vi "控件拖动.vi"() -> ()   [LabVIEW 2016]
uses:
  <vilib>/Utility/miscctls.llb/LVPointTypeDef.ctl
  <vilib>/Utility/miscctls.llb/LVPositionTypeDef.ctl
panel:
  in  "供电模块":T1 {"蓄电池2"."电量" format="%.0f %"; "蓄电池2"."电池电量" scale=0.0..100.0; "蓄电池2"."电流" format="%#.2g"; "蓄电池2"."电压" format="%#.2g"; "蓄电池"."电量" format="%.0f %"; "蓄电池"."电池电量" scale=0.0..100.0; "蓄电池"."电流" format="%#.2g"; "蓄电池"."电压" format="%#.2g"; "UPS"."电量" format="%.0f %"; "UPS"."电池电量" scale=0.0..100.0}
  out "拖动":bool
  in  "滑动杆":i32(slide) scale=-1000.0..1000.0
  # "V"
  # "A"
  # "V"
  # "A"
  # "V"
  # "V"
  # "V"
  # "A"
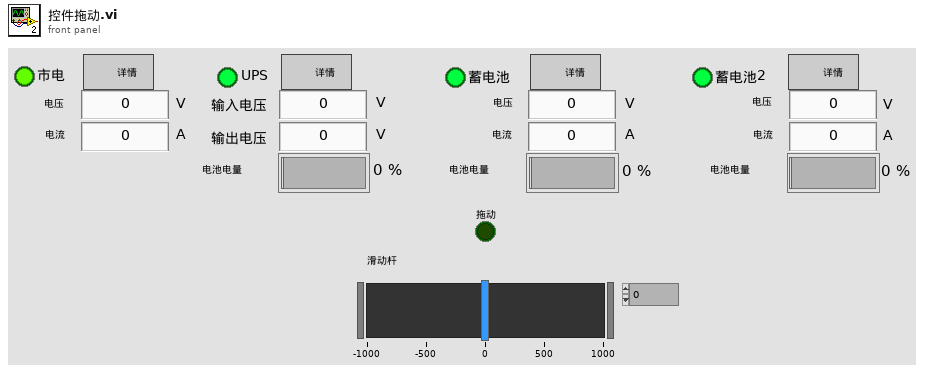
[diagram p1: front panel]
types:
  T1 = cluster{"市电":cluster{"市电":bool, "电压":u16, "电流":dbl, "市电监测":bool}, "UPS":cluster{"UPS":bool, "输入电压":sgl, "输出电压":sgl, "电池电量":u8, "电量":u16, "UPS监测":bool}, "蓄电池":cluster{"蓄电池":bool, "电压":sgl, "电流":sgl, "电池电量":u8, "电量":u16, "蓄电池监测":bool}, "蓄电池2":cluster{"蓄电池2":bool, "电压":sgl, "电流":sgl, "电池电量":u8, "电量":u16, "蓄电池监测2":bool}}
  T2 = typedef "LVPositionTypeDef.ctl" = cluster{"Left":i32, "Top":i32}
  T3 = typedef "LVPointTypeDef.ctl" = cluster{"Horizontal":i16, "Vertical":i16}
  T4 = typedef "LVPoint32TypeDef.ctl" = cluster{"Horizontal":i32, "Vertical":i32}
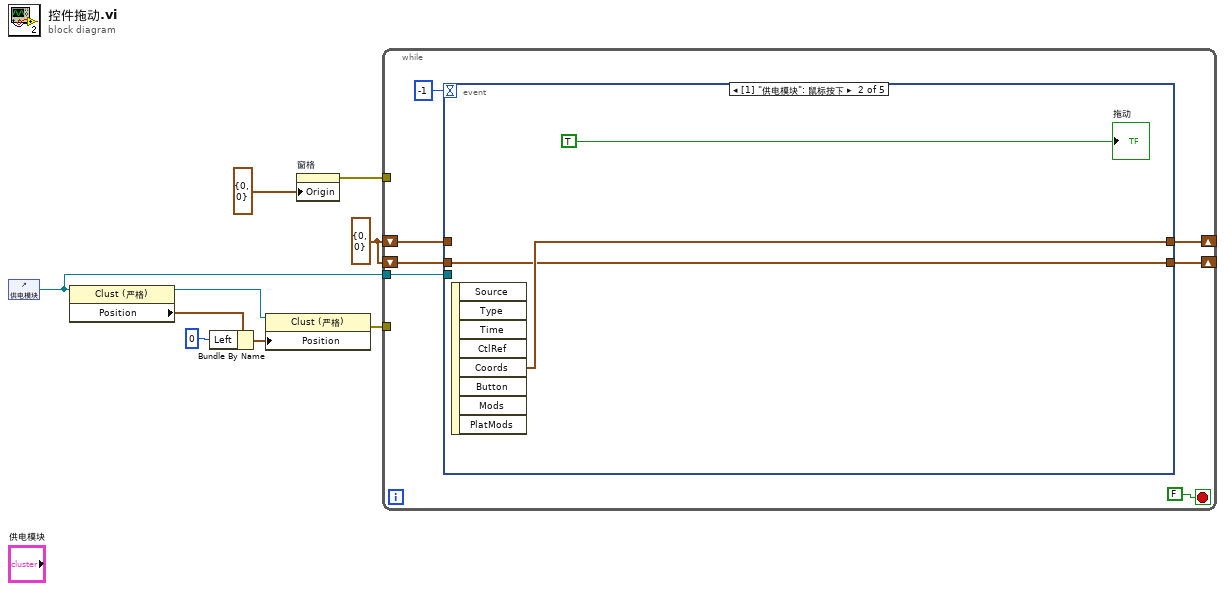
[diagram p0: block diagram]
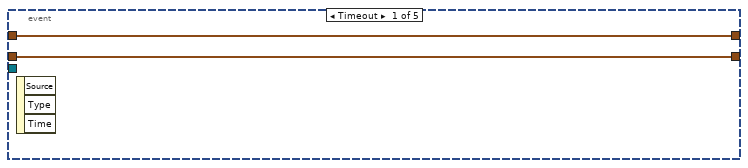
[diagram p2: hidden frame]
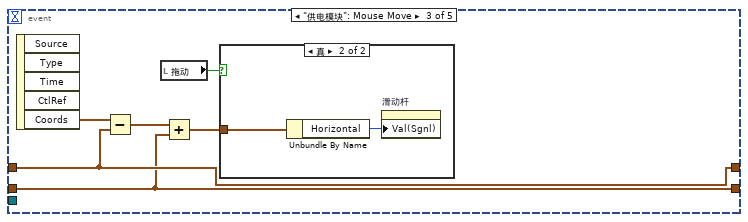
[diagram p3: hidden frame]
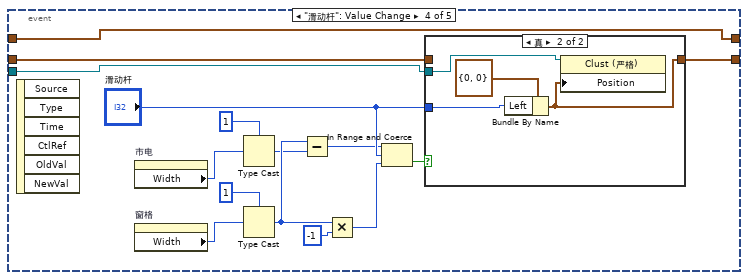
[diagram p5: hidden frame]
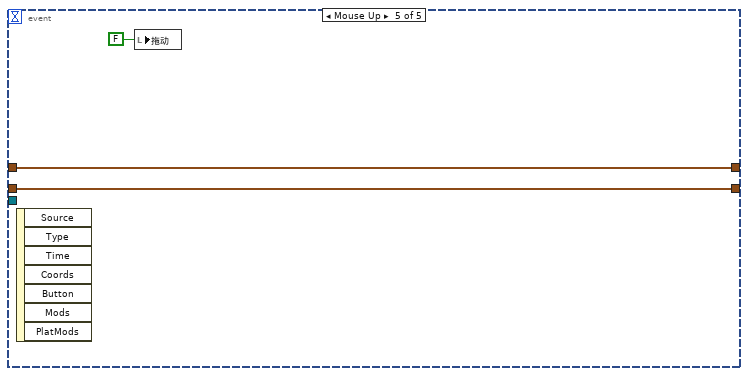
[diagram p7: hidden frame]
diagram:
  w6 = T2 {"Left"=0, "Top"=0} ("位置")
  n1 = control-ref of="供电模块"() -> (w1:refnum<vi>)
  n2 = property class="Clust (严格)"(reference=w1) -> (reference out=w3:refnum<vi>, "Position"=w4:T2)  [unwired: 1 in, 1 out]
  n3 = Bundle By Name(cluster=w4, "Left"=0) -> (w2:T2)
  n4 = property class="Clust (严格)"(reference=w3, "Position"=w2) -> (error out=w5:errorcluster)  [unwired: 1 in, 1 out]
  n5 = property on="窗格" class="Pane"("Origin"=T3 {"Horizontal"=0, "Vertical"=0} ("原点")) -> (error out=w8:errorcluster)  [unwired: 2 in, 1 out]
  n6 = while {
    tunnel: w8 -> [_]
    shift-right: [w14] -> _
    shift-left: w6 -> [w13]
    shift-right: [w12] -> _
    shift-left: w6 -> [w11]
    tunnel: w5 -> [_]
    tunnel: w1 -> [w10]
    stop <- FALSE stop-if-true
    n7 = event shown="[1] \"供电模块\": 鼠标按下" {
      selector: _ -> [_ _ _ _ _]
      dyn-events: _ -> [_ _ _ _ _]
      timeout: -1 -> [_ _ _ _ _]
      tunnel: [w17 w20 w27 w44 w51] -> w14
      tunnel: w13 -> [w17 _ w27 w44 w51]
      tunnel: [w18 w19 w25 w43 w50] -> w12
      tunnel: w11 -> [w18 w19 w25 w38 w50]
      tunnel: w10 -> [_ _ _ w30 _]
      event Timeout {
        n8 = event-data() -> ()  [unwired: 1 in, 3 out]
      }
      event "供电模块": Mouse Down {
        n9 = event-data() -> ("Coords"=w20:T4)  [unwired: 1 in, 7 out]
        "拖动" <- TRUE ("非x？")
      }
      event "供电模块": Mouse Move {
        n10 = event-data() -> ("Coords"=w26:T4)  [unwired: 1 in, 4 out]
        n11 = Subtract(x=w26, y=w27) -> (x-y=w24:T4)
        n12 = local read "拖动"() -> (w22:bool)
        n13 = Add(x=w24, y=w25) -> (x+y=w23:T4)
        n14 = case shown="真" w22 {
          tunnel: w23 -> [_ w28]
          frame False {
          }
          frame True {
            n15 = Unbundle By Name(w28) -> ("Horizontal"=w29:i32)
            n16 = property on="滑动杆" class="Slide (严格)"("Val(Sgnl)"=w29) -> ()  [unwired: 2 in, 2 out]
          }
        }
      }
      event "滑动杆": Value Change {
        n17 = event-data() -> ()  [unwired: 1 in, 6 out]
        n18 = property on="市电" class="Clust (严格)"() -> ("Width"=w32:u32)  [unwired: 2 in, 2 out]
        n19 = property on="窗格" class="Pane"() -> ("Width"=w36:u32)  [unwired: 2 in, 2 out]
        n20 = Type Cast(type=1 ("y"), x=w32) -> (*(type *) &x=w31:i32)
        n21 = Type Cast(type=1 ("y"), x=w36) -> (*(type *) &x=w35:i32)
        n22 = Subtract(x=w35, y=w31) -> (x-y=w34:i32)
        n23 = Multiply(x=w35, y=-1) -> (x*y=w40:i32)
        n24 = In Range and Coerce(upper limit=w34, x="滑动杆", lower limit=w40) -> (In Range?=w39:bool)  [unwired: 1 out]
        n25 = case shown="真" w39 {
          tunnel: [w45 w47] -> w43
          tunnel: "滑动杆" -> [_ w48]
          tunnel: w38 -> [w45 _]
          tunnel: w30 -> [_ w46]
          frame False {
          }
          frame True {
            n26 = Bundle By Name(cluster=T2 {"Left"=0, "Top"=0} ("位置"), "Left"=w48) -> (w47:T2)
            n27 = property class="Clust (严格)"(reference=w46, "Position"=w47) -> ()  [unwired: 1 in, 2 out]
          }
        }
      }
      event Mouse Up {
        n28 = event-data() -> ()  [unwired: 1 in, 7 out]
        n29 = local write "拖动"(FALSE ("非x？")) -> ()
      }
    }
  }
